vi "CRYDigital IO H Port Convert.vi"(10 "In Data":u8) -> (2 "Out Data":u8)   [LabVIEW 2013]
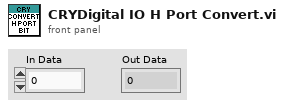
[diagram p1: front panel]
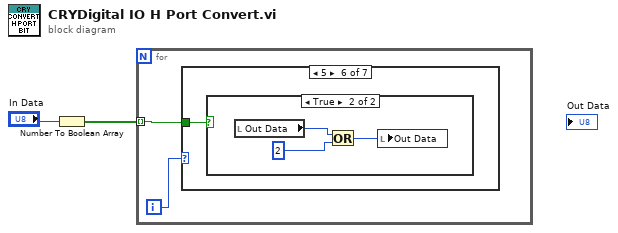
[diagram p0: block diagram]
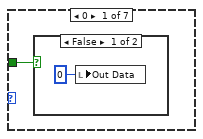
[diagram p2: hidden frame]
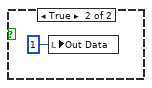
[diagram p3: hidden frame]
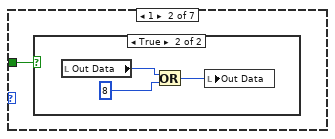
[diagram p4: hidden frame]
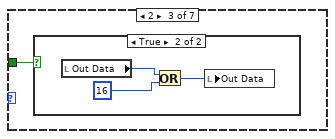
[diagram p6: hidden frame]
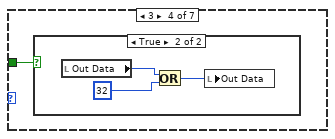
[diagram p8: hidden frame]
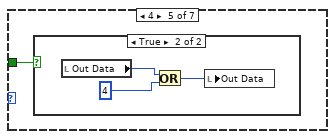
[diagram p10: hidden frame]
diagram:
  n1 = Number To Boolean Array(number="In Data") -> (Boolean array=w1:bool[])
  n2 = for {
    tunnel: w1 -> [w3] mode=indexing
    i -> [w4]
    n3 = case shown="5" w4 {
      tunnel: w3 -> [w5 w8 w12 w16 w20 w24 _]
      frame 0 {
        n4 = case shown="False" w5 {
          frame False {
            n5 = local write "Out Data"(u8 0 ("Out Data")) -> ()
          }
          frame True {
            n6 = local write "Out Data"(u8 1 ("Out Data")) -> ()
          }
        }
      }
      frame 1 {
        n7 = case shown="True" w8 {
          frame False {
          }
          frame True {
            n8 = local read "Out Data"() -> (w11:u8)
            n9 = Or(x=w11, y=u8 8) -> (x .or. y?=w9:u8)
            n10 = local write "Out Data"(w9) -> ()
          }
        }
      }
      frame 2 {
        n11 = case shown="True" w12 {
          frame False {
          }
          frame True {
            n12 = local read "Out Data"() -> (w15:u8)
            n13 = Or(x=w15, y=u8 16) -> (x .or. y?=w13:u8)
            n14 = local write "Out Data"(w13) -> ()
          }
        }
      }
      frame 3 {
        n15 = case shown="True" w16 {
          frame False {
          }
          frame True {
            n16 = local read "Out Data"() -> (w19:u8)
            n17 = Or(x=w19, y=u8 32) -> (x .or. y?=w17:u8)
            n18 = local write "Out Data"(w17) -> ()
          }
        }
      }
      frame 4 {
        n19 = case shown="True" w20 {
          frame False {
          }
          frame True {
            n20 = local read "Out Data"() -> (w23:u8)
            n21 = Or(x=w23, y=u8 4) -> (x .or. y?=w21:u8)
            n22 = local write "Out Data"(w21) -> ()
          }
        }
      }
      frame 5 {
        n23 = case shown="True" w24 {
          frame False {
          }
          frame True {
            n24 = local read "Out Data"() -> (w27:u8)
            n25 = Or(x=w27, y=u8 2) -> (x .or. y?=w25:u8)
            n26 = local write "Out Data"(w25) -> ()
          }
        }
      }
      frame Default {
      }
    }
  }
